vi "Camera Main.vi"(8 "Timeout 2":refnum<vi>, 9 "Main Open and Save Ctrls Ref":refnum<vi>[](array[refnum]), 11 "Camera":string) -> ()   [LabVIEW 2025]
uses:
  Camera Set Up/Ctrl/White Balance.ctl
  <vilib>/Utility/sysdir.llb/System Directory Type.ctl
  Main State Machine/Ctrl's/Main Cluster.ctl
  Main State Machine/Ctrl's/Main Queue.ctl
  Main State Machine/Ctrl's/Main States.ctl
  <vilib>/userDefined/High Color/IMAQdx.ctl
  <vilib>/vision/Image Controls.llb/IMAQ Image.ctl
  Camera Set Up/Event/Event Setup Types.ctl
  41b0be78-b641-410b-9a45-cddc263d6dc9.vi
  <vilib>/Utility/config.llb/Read Key (String).vi
  <vilib>/Utility/config.llb/Write Key (String).vi
  <vilib>/regexp/Match Regular Expression.xnode
  <vilib>/vision/driver/NI_Vision_Acquisition_Software.lvlib
  <vilib>/Utility/config.llb/NI_LVConfig.lvlib
  <resource>/objmgr/imaqdx.rc
  <vilib>/vision/NI_Vision_Development_Module.lvlib
panel:
  in  "Main":enum32{"Camera Settings", "Camera Settings 2"}(tab)
  out "Title":string="cam0"
  out "Greyscale":bool
  out "Camera Image":T1(plugin-control)
  in  "Save 2":bool caption="Save"
  in  "Reset Camera":bool
  in  "VideoMode":u16(ring)=20 items=["640x360 MJPG 260.00fps", "1280x720 MJPG 120.00fps", "1920x1080 MJPG 60.00fps"]
  in  "Saturation":i32(slide)=50 min=0 max=100 scale=0.0..100.0
  in  "Hue":i32(slide)=50 min=0 max=100 scale=0.0..100.0
  in  "Gamma":i32(slide)=50 min=0 max=100 scale=0.0..100.0
  in  "Exposure":dbl(slide)=2.0 min=0.0 max=100.0 step=0.01 scale=0.0..100.0
  in  "Contrast":i32(slide)=50 min=0 max=100 scale=0.0..100.0
  in  "Sharpness":i32(slide)=50 min=0 max=100 scale=0.0..100.0
  in  "White Balance":T2=enum."Hold current"
  in  "Gain":i32(slide)=50 min=0 max=100 scale=0.0..100.0
  in  "Brightness":i32(slide)=50 min=0 max=100 scale=0.0..100.0
  out "Width 2":u32=640 caption="Width"
  out "Height 2":u32=360 caption="Height"
  out "Processed FPS":dbl format="%.1f"
  out "Acquired FPS":dbl format="%.1f"
  out "Timeout":u32
  out "Running":bool
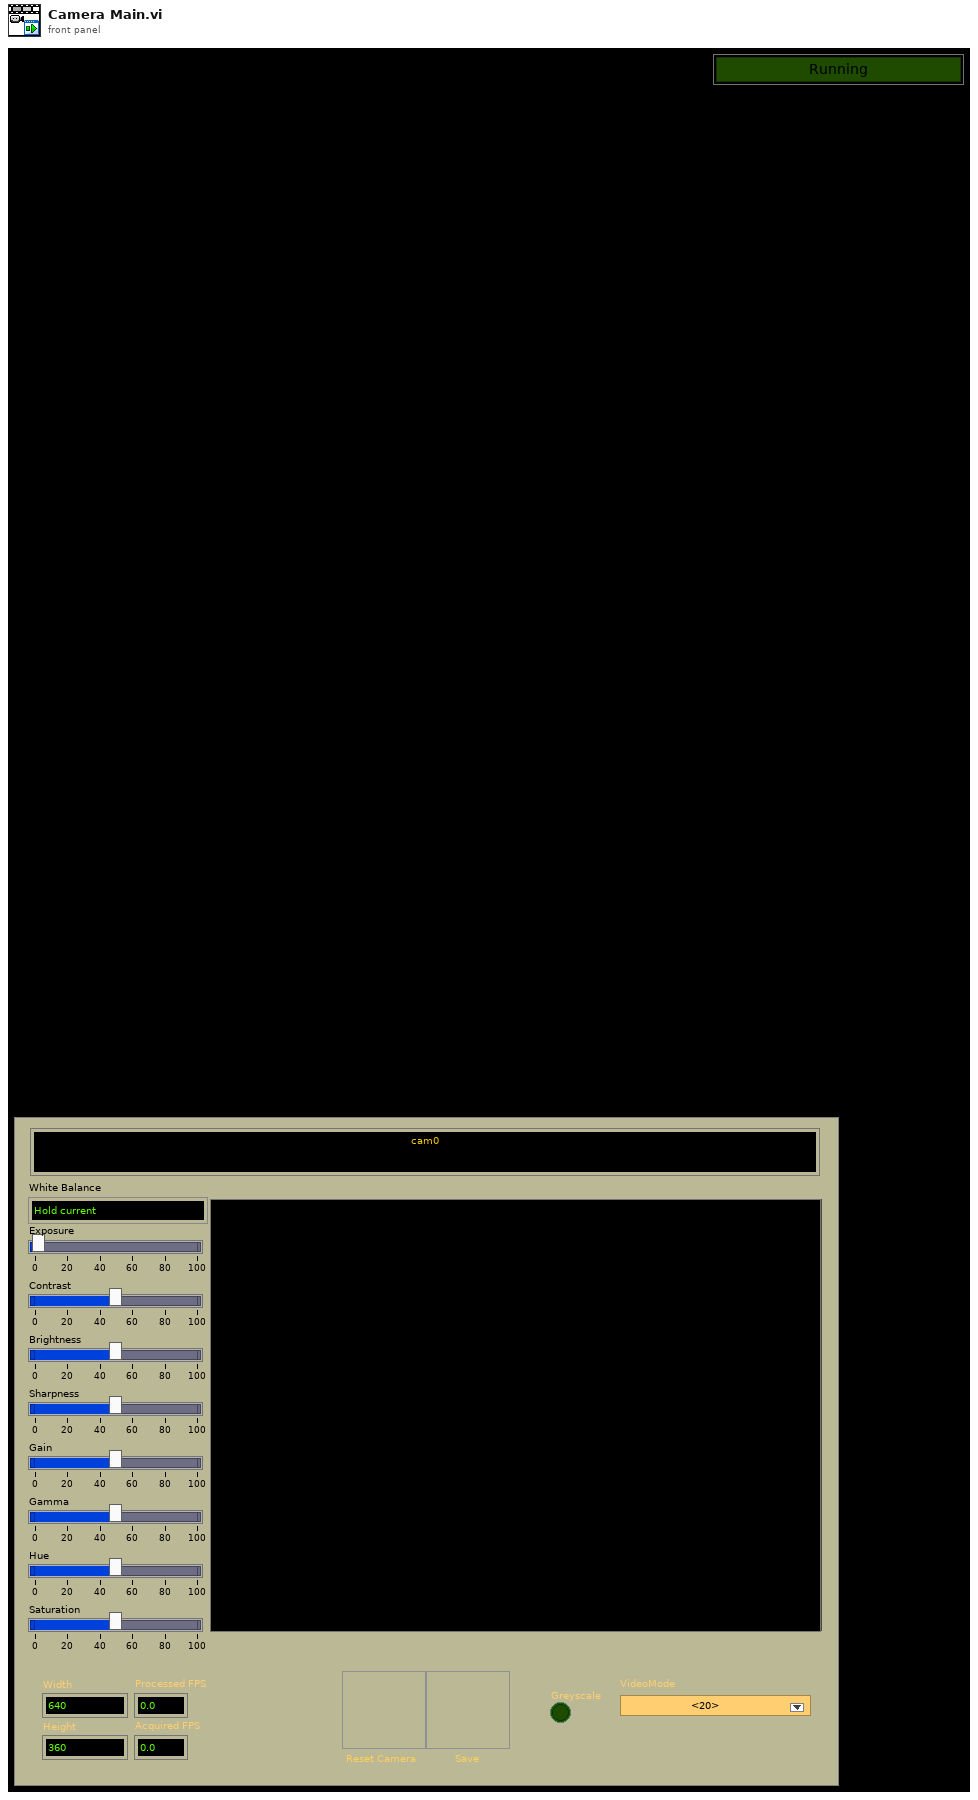
[diagram p1: front panel]
types:
  T1 = typedef "IMAQ Image.ctl" = refnum<image>
  T2 = typedef "White Balance.ctl" = enum16{"Auto", "Fixed indoor", "Fixed outdoor 1", "Fixed outdoor 2", "Fixed fluorescent 1", "Fixed fluorescent 2", "Hold current", "Custom"}
  T3 = typedef "System Directory Type.ctl" = i32
  T4 = typedef "Image Type" = u32
  T5 = typedef "Main Cluster.ctl" = cluster{"Main Queue":T6, "error":errorcluster, "Camera":T8, "Camera Session":T8, "Image In":T1, "White Balance":T2, "Attr String":string[], "Values":dbl[], "VideoMode":u16, "Exposure":i32, "Reset":bool, "Greyscale":bool, "INI path":path, "Default path":path, "INI File Found":bool, "Open And Save Controls":refnum<vi>[], "Buffer":u32, "Main Timeout ref":refnum<vi>, "Main Open and Save Ctrls Ref":refnum<vi>[]}
  T6 = typedef "Main Queue.ctl" = T7[]
  T7 = typedef "Main States.ctl" = enum16{"Message Dispatcher", "INI", "End Session", "Camera Process Settings", "Camera Open Default", "Camera Save Default", "Get Values", "Get VideoMode", "Open Camera", "Open Settings", "Save Settings", "Set Value", "Set VideoMode", "Set WB", "Setup Camera", "Start Session", "Exit"}
  T8 = typedef "IMAQdx.ctl" = refnum<k21>
  T9 = typedef "Event Setup Types.ctl" = enum16{"Default", "Camera Loop Started", "GreyScale", "Reset Camera Settings", "Reset Team Number", "Save Data", "Setting Changed", "Update Video Mode", "Video Mode Changed", "Exit"}
  T10 = enum8{"Enabled", "Disabled", "Disabled and Grayed Out"}
  T11 = typedef "NI_LVConfig.lvlib/Config Data RefNum.ctl" = refnum<k1>
  T12 = cluster{"Video Mode":u32, "Video Mode Name":string}[]
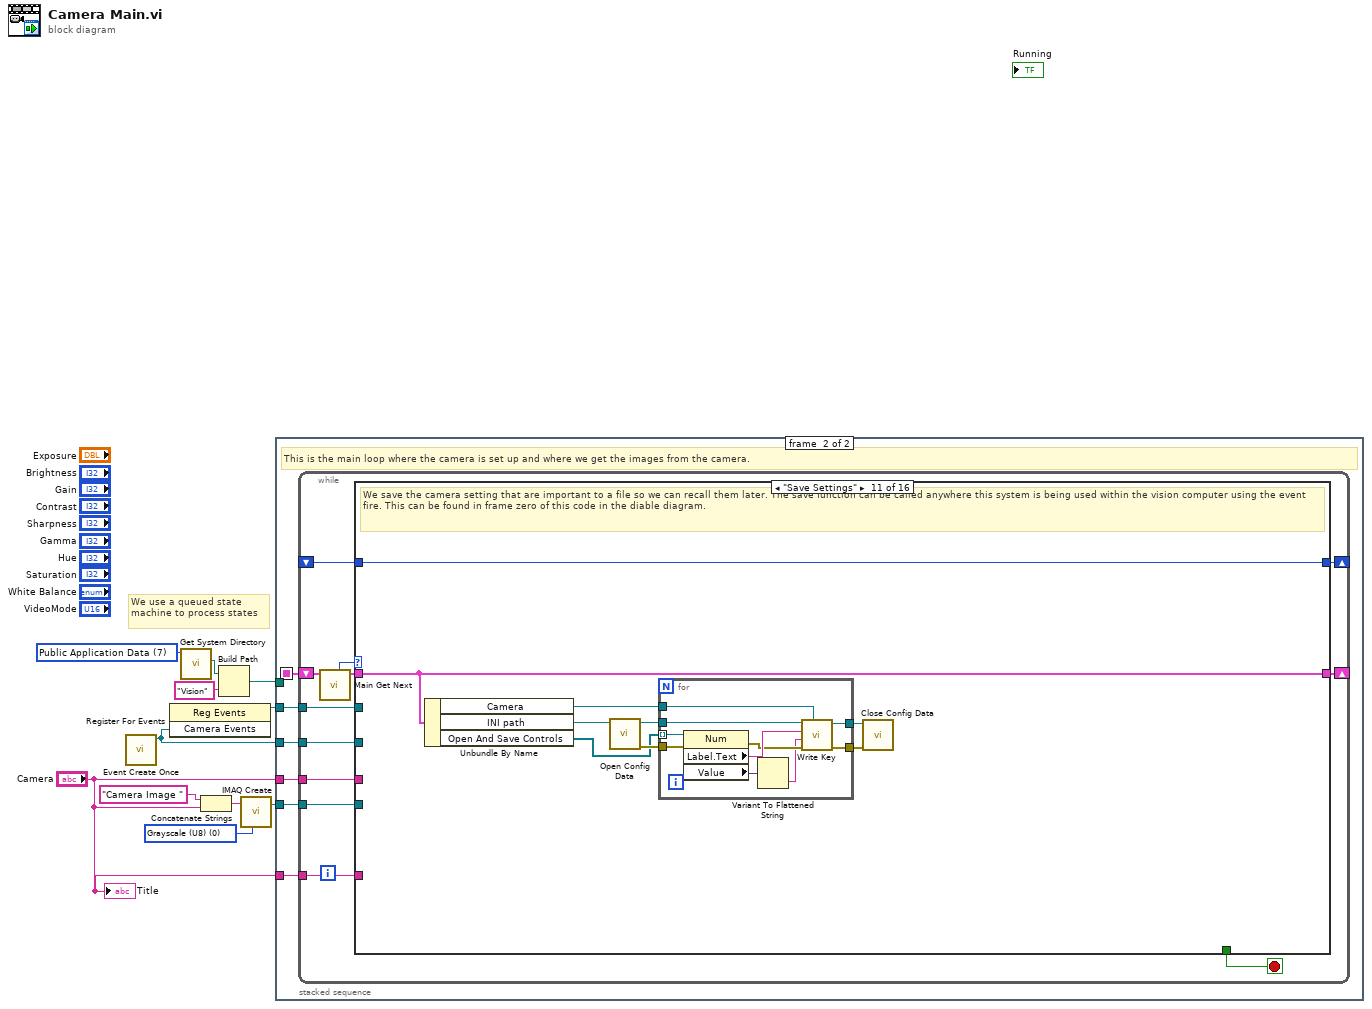
[diagram p0: block diagram]
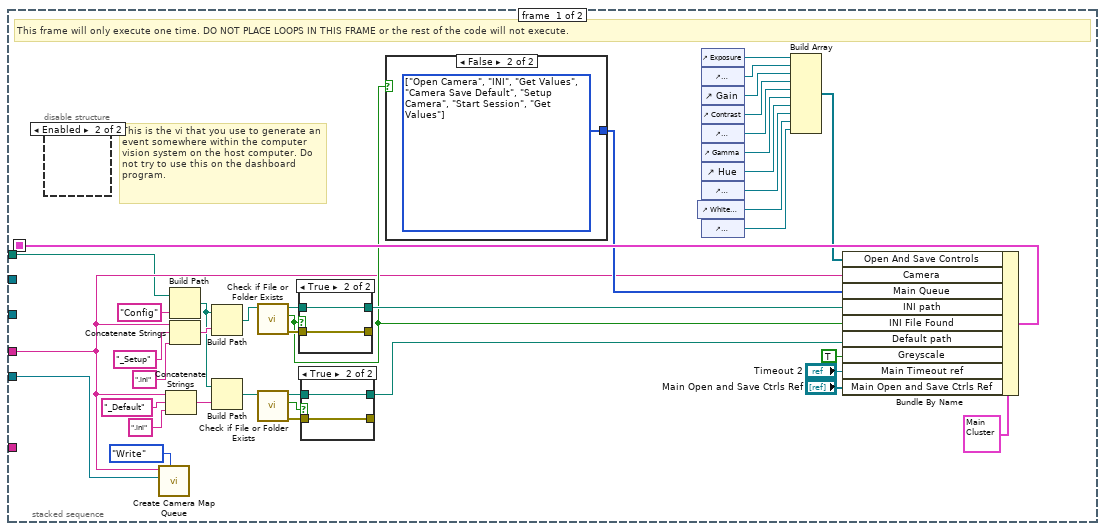
[diagram p2: hidden frame]
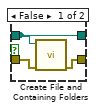
[diagram p3: hidden frame]
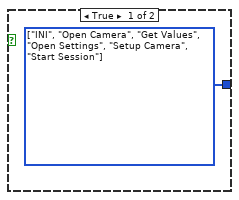
[diagram p4: hidden frame]
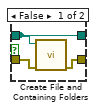
[diagram p5: hidden frame]
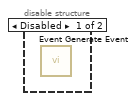
[diagram p6: hidden frame]
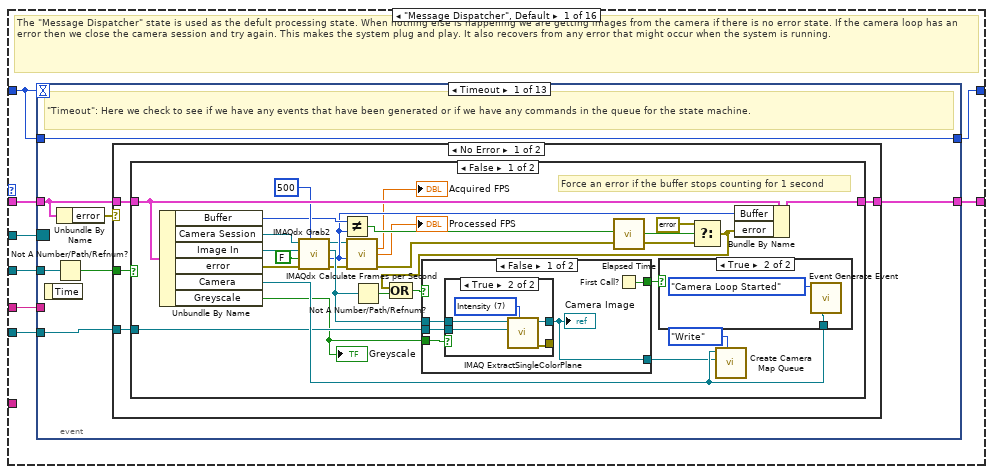
[diagram p7: hidden frame]
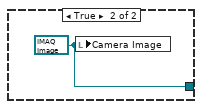
[diagram p10: hidden frame]
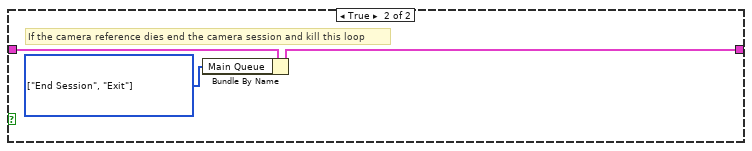
[diagram p11: hidden frame]
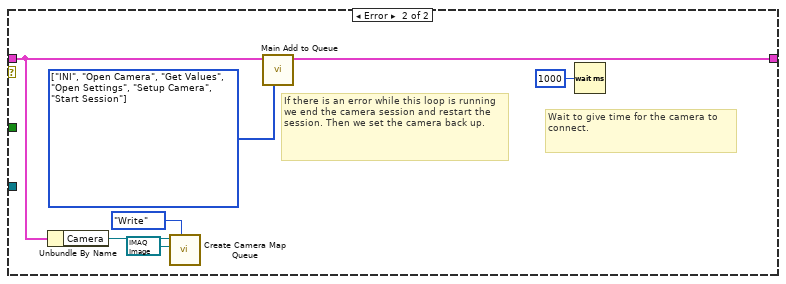
[diagram p12: hidden frame]
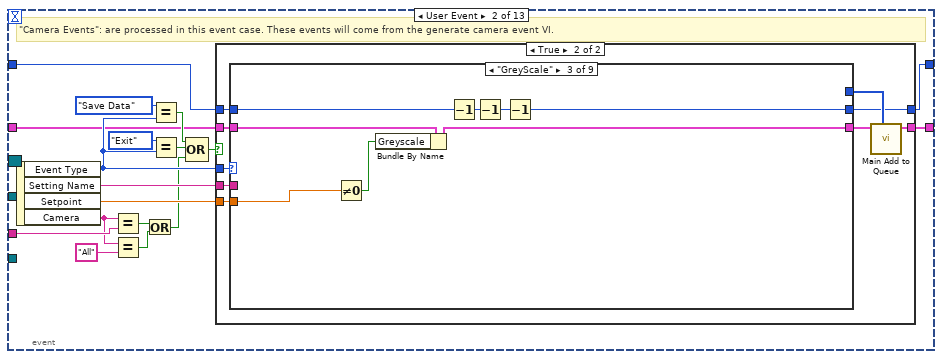
[diagram p13: hidden frame]
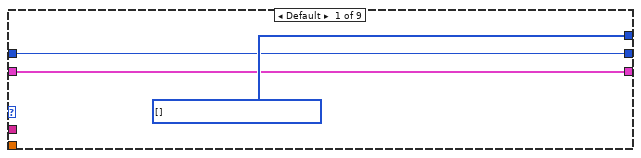
[diagram p15: hidden frame]
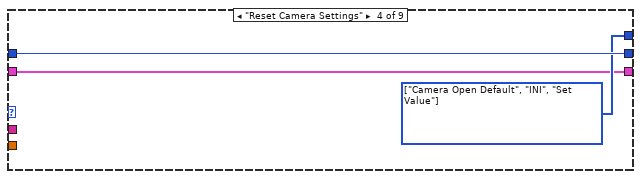
[diagram p17: hidden frame]
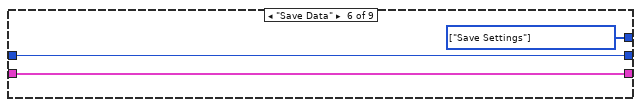
[diagram p19: hidden frame]
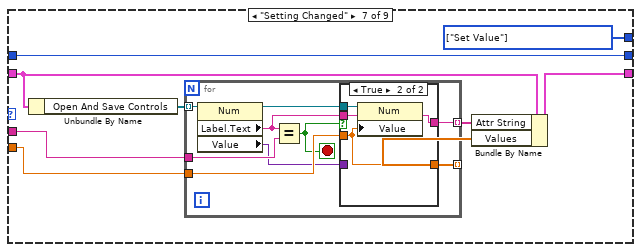
[diagram p20: hidden frame]
diagram:
  w5 = T3 7 items=["User Home"=0, "User Desktop"=1, "User Documents"=2, "User Application Data"=3, "User Preferences"=4, "User Temporary"=5, "Public Documents"=6, "Public Application Data"=7, "Public Preferences"=8, "Public Cache"=13, "System Core Libraries"=9, "System Installed Libraries"=10, "Application Files"=11, "Boot Volume Root"=12] ("system directory type")
  w8 = T4 0 items=["Grayscale (U8)", "Grayscale (I16)", "Grayscale (SGL)", "Complex (CSG)", "RGB (U32)", "HSL (U32)", "RGB (U64)", "Grayscale (U16)"] ("Image Type")
  # "We use a queued state machine to process states"
  n1 = call "Event Create Once.vi"() -> ("Camera Events"=w6:refnum<user-event>)  [unwired: 10 in, 1 out]
  n2 = register-events(w6) -> (reference out=w11:refnum<event-registration>)  [unwired: 2 in, 1 out]
  n3 = call <vilib>:"Get System Directory.vi"("system directory type"=w5) -> ("system directory"=w4:path)  [unwired: 10 in]
  n4 = Concatenate Strings("Camera Image " ("string"), "Camera") -> (w10:string)
  n5 = Build Path(base path=w4, name or relative path="Vision") -> (appended path=w3:path)
  n6 = call "IMAQ Create"("Image Name"=w10, "Image Type"=w8) -> ("New Image"=w7:T1)  [unwired: 2 in, 2 out]
  n7 = stacked-sequence {
    seq-local: [w46 _] -> [_ w68]
    tunnel: w11 -> [_ w67]
    tunnel: w6 -> [_ w66]
    tunnel: "Camera" -> [w25 w65]
    tunnel: w7 -> [w26 w64]
    tunnel: w3 -> [w13 _]
    tunnel: "Camera" -> [_ w63]
    frame #0 {
      # "This is the vi that you use to generate an event somewhere within the computer vision system on the host computer. Do not try to use this on the dashboard program."
      # "This frame will only execute one time. DO NOT PLACE LOOPS IN THIS FRAME or the rest of the code will not execute."
      n8 = disable-structure shown="Enabled" {
        frame Disabled {
          n9 = call "Event Generate Event.vi"() -> ()  [unwired: 12 in]
        }
        frame Enabled {
        }
      }
      n10 = call "Create Camera Map Queue.vi"("Action"=enum16{"Read", "Write"}."Write", "Image in"=w26, "Camera"=w25) -> ()  [unwired: 7 in, 2 out]
      n11 = Concatenate Strings(w25, "_Default" ("string"), ".ini" ("name or relative path")) -> (w28:string)
      n12 = Build Path(base path=w13, name or relative path="Config") -> (appended path=w31:path)
      n13 = Concatenate Strings(w25, "_Setup" ("string"), ".ini" ("name or relative path")) -> (w49:string)
      n14 = Build Path(base path=w31, name or relative path=w49) -> (appended path=w44:path)
      n15 = Build Path(base path=w31, name or relative path=w28) -> (appended path=w33:path)
      n16 = call <vilib>:"Check if File or Folder Exists.vi"("path"=w44) -> ("error out"=w45:errorcluster, "file or folder exists?"=w37:bool, "dup path"=w43:path)  [unwired: 8 in]
      n17 = call <vilib>:"Check if File or Folder Exists.vi"("path"=w33) -> ("error out"=w36:errorcluster, "file or folder exists?"=w34:bool, "dup path"=w35:path)  [unwired: 8 in]
      n18 = case shown="True" w37 {
        tunnel: [w60 w61] -> _
        tunnel: w45 -> [w59 w61]
        tunnel: w43 -> [w58 w62]
        tunnel: [w58 w62] -> w42
        frame False {
          n19 = call <vilib>:"Create File and Containing Folders.vi"("error in (no error)"=w59, "file path"=w58) -> ("error out"=w60:errorcluster)  [unwired: 8 in, 1 out]
        }
        frame True {
        }
      }
      n20 = case shown="True" w34 {
        tunnel: [w53 w54] -> _
        tunnel: w36 -> [w52 w54]
        tunnel: w35 -> [w51 w55]
        tunnel: [w51 w55] -> w32
        frame False {
          n21 = call <vilib>:"Create File and Containing Folders.vi"("error in (no error)"=w52, "file path"=w51) -> ("error out"=w53:errorcluster)  [unwired: 8 in, 1 out]
        }
        frame True {
        }
      }
      n22 = case shown="False" w37 {
        tunnel: [w56 w57] -> w38
        frame True {
          w56 = T6 [enum."INI", enum."Open Camera", enum."Get Values", enum."Open Settings", enum."Setup Camera", enum."Start Session"] items=["Message Dispatcher", "INI", "End Session", "Camera Process Settings", "Camera Open Default", "Camera Save Default", "Get Values", "Get VideoMode", "Open Camera", "Open Settings", "Save Settings", "Set Value", "Set VideoMode", "Set WB", "Setup Camera", "Start Session", "Exit"] ("Main Queue")
        }
        frame False {
          w57 = T6 [enum."Open Camera", enum."INI", enum."Get Values", enum."Camera Save Default", enum."Setup Camera", enum."Start Session", enum."Get Values"] items=["Message Dispatcher", "INI", "End Session", "Camera Process Settings", "Camera Open Default", "Camera Save Default", "Get Values", "Get VideoMode", "Open Camera", "Open Settings", "Save Settings", "Set Value", "Set VideoMode", "Set WB", "Setup Camera", "Start Session", "Exit"] ("Main Queue")
        }
      }
      n23 = control-ref of="White Balance"() -> (w15:refnum<vi>)
      n24 = control-ref of="Exposure"() -> (w23:refnum<vi>)
      n25 = control-ref of="Brightness"() -> (w22:refnum<vi>)
      n26 = control-ref of="Gain"() -> (w21:refnum<vi>)
      n27 = control-ref of="Contrast"() -> (w20:refnum<vi>)
      n28 = control-ref of="Sharpness"() -> (w19:refnum<vi>)
      n29 = control-ref of="Gamma"() -> (w18:refnum<vi>)
      n30 = control-ref of="Hue"() -> (w17:refnum<vi>)
      n31 = control-ref of="Saturation"() -> (w16:refnum<vi>)
      n32 = control-ref of="VideoMode"() -> (w14:refnum<vi>)
      n33 = Build Array(w23, w22, w21, w20, w19, w18, w17, w16, w15, w14) -> (w41:refnum<vi>[])
      n34 = Bundle By Name(cluster=T5 {"Main Queue"=[], "error"={"status"=FALSE, "code"=0, "source"=""}, "Camera"="", "Camera Session"="", "Image In"=refnum, "White Balance"=enum."Hold current", "Attr String"=[], "Values"=[], "VideoMode"=0, "Exposure"=50, "Reset"=FALSE, "Greyscale"=FALSE, "INI path"=path "", "Default path"=path "", "INI File Found"=FALSE, "Open And Save Controls"=[], "Buffer"=0, "Main Timeout ref"=refnum, "Main Open and Save Ctrls Ref"=[]} ("Main Cluster Out"), "Open And Save Controls"=w41, "Camera"=w25, "Main Queue"=w38, "INI path"=w42, "INI File Found"=w37, "Default path"=w32, "Greyscale"=TRUE, "Main Timeout ref"="Timeout 2", "Main Open and Save Ctrls Ref"="Main Open and Save Ctrls Ref") -> (w46:T5)
    }
    frame #1 {
      # "This is the main loop where the camera is set up and where we get the images from the camera."
      n35 = while {
        shift-right: [w76] -> _
        shift-left: w68 -> [w78]
        tunnel: w67 -> [w75]
        shift-right: [w74] -> _
        shift-left: _ -> [w73]
        tunnel: w66 -> [w72]
        tunnel: w65 -> [w71]
        tunnel: w64 -> [w70]
        tunnel: w63 -> [w69]
        stop <- w80 stop-if-true
        n36 = call "Main Get Next.vi"("Main Cluster In"=w78) -> ("Main Cluster Out"=w77:T5, "Next State"=w79:T7)  [unwired: 9 in]
        n37 = case shown="\"Save Settings\"" w79 {
          tunnel: [_ _ _ _ _ _ _ _ _ _ _ _ _ _ _ TRUE] -> w80
          tunnel: w77 -> [w87 w327 w339 w347 w390 w395 w417 w465 w591 w610 w658 w677 w695 w754 w890 w899]
          tunnel: [w88 w328 w336 w344 w388 w395 w416 w464 w590 w606 w658 w676 w705 w752 w884 w899] -> w76
          tunnel: w75 -> [w86 _ _ _ _ _ _ _ _ _ _ _ _ _ _ _]
          tunnel: w73 -> [w84 w330 w337 w351 w389 w400 w422 _ w596 w614 w663 w683 w694 _ w887 w897]
          tunnel: [w83 w330 w337 w351 w389 w400 w422 w439 w596 w614 w663 w683 w694 w728 w887 w897] -> w74
          tunnel: w72 -> [w85 _ _ _ _ _ _ _ _ _ _ _ _ _ _ _]
          tunnel: w71 -> [w82 _ _ _ _ _ _ _ _ _ _ _ _ _ _ _]
          tunnel: w70 -> [w81 _ _ _ _ _ _ _ _ _ _ _ _ _ _ _]
          tunnel: w69 -> [_ _ _ _ _ _ _ _ w585 _ _ _ _ _ _ _]
          frame "Message Dispatcher", Default {
            # "The \"Message Dispatcher\" state is used as the defult processing state. When nothing else is happening we are getting images from the camera if there is no error state. If the camera loop has an error then we close the camera session and try again. This makes the system plug and play. It also recovers from any error that might occur when the system is running."
            n38 = event shown="[0] Timeout" {
              selector: w86 -> [_ _ _ _ _ _ _ _ _ _ _ _ _]
              dyn-events: _ -> [_ _ _ _ _ _ _ _ _ _ _ _ _]
              timeout: w84 -> [_ _ _ _ _ _ _ _ _ _ _ _ _]
              tunnel: [w95 w168 w240 w250 w260 w270 w280 w284 w291 w298 w308 w314 w323] -> w88
              tunnel: w87 -> [w94 w161 w242 w252 w262 w272 w282 w287 w290 w300 w310 w316 w325]
              tunnel: w85 -> [w92 _ _ _ _ _ _ _ _ _ _ _ _]
              tunnel: w84 -> [w90 w160 w234 w244 w254 w264 w274 w285 w288 w292 w302 w312 w321]
              tunnel: [w90 w159 w234 w244 w254 w264 w274 w285 w288 w292 w302 w312 w321] -> w83
              tunnel: w82 -> [_ w158 _ _ _ _ _ _ _ _ _ _ _]
              tunnel: w81 -> [w89 _ _ _ _ _ _ _ _ _ _ _ _]
              event Timeout {
                # "\"Timeout\": Here we check to see if we have any events that have been generated or if we have any commands in the queue for the state machine."
                n39 = event-data() -> ()  [unwired: 1 in, 1 out]
                n40 = Not A Number/Path/Refnum?(number/path/refnum=w92) -> (NaN/Path/Refnum?=w91:bool)
                n41 = Unbundle By Name(w94) -> ("error"=w93:errorcluster)
                n42 = case shown="No Error" w93 {
                  tunnel: w94 -> [w99 w147]
                  tunnel: [w98 w150] -> w95
                  tunnel: w91 -> [w97 _]
                  tunnel: w89 -> [w96 _]
                  frame No Error {
                    n43 = case shown="False" w97 {
                      tunnel: w99 -> [w126 w143]
                      tunnel: [w121 w142] -> w98
                      tunnel: w96 -> [w119 _]
                      frame False {
                        # "Force an error if the buffer stops counting for 1 second"
                        n44 = Unbundle By Name(w126) -> ("Buffer"=w107:u32, "Camera Session"=w106:T8, "Image In"=w125:T1, "error"=w124:errorcluster, "Camera"=w122:T8, "Greyscale"=w118:bool)
                        "Greyscale" <- w118
                        n45 = call <vilib>:"IMAQdx Grab2.vi"("Timeout (ms)"=500, "error in"=w124, "Wait for Next Buffer? (Yes)"=FALSE, "Image In"=w125, "Session In"=w106) -> ("error out"=w102:errorcluster, "Buffer Number Out"=w105:u32, "Image Out"=w114:T1, "Session Out"=w100:T8)  [unwired: 3 in]
                        n46 = Not Equal?(x=w107, y=w105) -> (x != y?=w116:bool)
                        n47 = call <vilib>:"IMAQdx Calculate Frames per Second.vi"("Session In"=w100, "Buffer Number"=w105, "error in (no error)"=w102) -> ("Acquired Frames per Second"=→"Acquired FPS":dbl, "Processed Frames per Second"=→"Processed FPS":dbl, "error out"=w101:errorcluster)  [unwired: 6 in, 4 out]
                        n48 = Not A Number/Path/Refnum?(number/path/refnum=w114) -> (NaN/Path/Refnum?=w113:bool)
                        n49 = call "Elapsed Time"("Reset"=w116) -> ("Time has Elapsed"=w115:bool)  [unwired: 11 in, 7 out]
                        n50 = Select(t=errorcluster {"status"=TRUE, "code"=1, "source"=""}, s=w115, f=w101) -> (s? t:f=w112:errorcluster)
                        n51 = Compound Arithmetic op=OR(w112, w113) -> (w111:bool)
                        n52 = case shown="False" w111 {
                          tunnel: w114 -> [w132 _]
                          tunnel: [w133 _] -> w123
                          tunnel: w119 -> [w131 _]
                          tunnel: w118 -> [w130 _]
                          tunnel: [w129 w140] -> w109
                          frame False {
                            n53 = case shown="True" w130 {
                              tunnel: w132 -> [w134 w139]
                              tunnel: [w134 w138] -> w129
                              tunnel: w131 -> [_ w136]
                              tunnel: [_ w135] -> _
                              frame False {
                              }
                              frame True {
                                w137 = 7 items=["Red", "Green", "Blue", "Hue", "Saturation", "Luminance", "Value", "Intensity"] ("Color Plane")
                                n54 = call "IMAQ ExtractSingleColorPlane"("Color Plane"=w137, "Image Dst"=w136, "Image Src"=w139) -> ("error out"=w135:errorcluster, "Image Dst Out"=w138:T1)  [unwired: 7 in]
                              }
                            }
                            "Camera Image" <- w129
                            n55 = First Call?() -> (First Call?: T/F=w133:bool)
                          }
                          frame True {
                            w140 = T1 refnum ("Camera Image")
                            n56 = local write "Camera Image"(w140) -> ()
                          }
                        }
                        n57 = case shown="True" w123 {
                          tunnel: w122 -> [_ w127]
                          frame False {
                          }
                          frame True {
                            n58 = call "Event Generate Event.vi"("Camera Name"=w127, "Event Type"=Event_Setup_Types."Camera Loop Started") -> ()  [unwired: 10 in]
                          }
                        }
                        n59 = call "Create Camera Map Queue.vi"("Action"=enum16{"Read", "Write"}."Write", "Image in"=w109, "Camera"=w122) -> ()  [unwired: 7 in, 2 out]
                        n60 = Bundle By Name(cluster=w126, "Buffer"=w105, "error"=w112) -> (w121:T5)
                      }
                      frame True {
                        w141 = T6 [enum."End Session", enum."Exit"] items=["Message Dispatcher", "INI", "End Session", "Camera Process Settings", "Camera Open Default", "Camera Save Default", "Get Values", "Get VideoMode", "Open Camera", "Open Settings", "Save Settings", "Set Value", "Set VideoMode", "Set WB", "Setup Camera", "Start Session", "Exit"] ("Main Queue")
                        # "If the camera reference dies end the camera session and kill this loop"
                        n61 = Bundle By Name(cluster=w143, "Main Queue"=w141) -> (w142:T5)
                      }
                    }
                  }
                  frame Error {
                    w144 = T6 [enum."INI", enum."Open Camera", enum."Get Values", enum."Open Settings", enum."Setup Camera", enum."Start Session"] items=["Message Dispatcher", "INI", "End Session", "Camera Process Settings", "Camera Open Default", "Camera Save Default", "Get Values", "Get VideoMode", "Open Camera", "Open Settings", "Save Settings", "Set Value", "Set VideoMode", "Set WB", "Setup Camera", "Start Session", "Exit"] ("Main Queue")
                    # "Wait to give time for the camera to connect."
                    # "If there is an error while this loop is running we end the camera session and restart the session. Then we set the camera back up."
                    n62 = Unbundle By Name(w147) -> ("Camera"=w146:T8)
                    n63 = call "Create Camera Map Queue.vi"("Action"=enum16{"Read", "Write"}."Write", "Image in"=T1 refnum, "Camera"=w146) -> ()  [unwired: 7 in, 2 out]
                    n64 = call "Main Add to Queue.vi"("Main Queue"=w144, "Main Cluster In"=w147) -> ("Main Cluster Out"=w150:T5)  [unwired: 9 in]
                    n65 = Wait (ms)(milliseconds to wait=u32 1000) -> ()  [unwired: 1 out]
                  }
                }
              }
              event User Event {
                # "\"Camera Events\": are processed in this event case. These events will come from the generate camera event VI."
                n66 = event-data() -> ("Event Type"=w162:T9, "Setting Name"=w157:string, "Setpoint"=w156:dbl, "Camera"=w153:string)  [unwired: 1 in]
                n67 = Equal?(x=w153, y=w158) -> (x = y?=w154:bool)
                n68 = Equal?(x=w153, y="All") -> (x = y?=w151:bool)
                n69 = Or(x=w154, y=w151) -> (x .or. y?=w155:bool)
                n70 = Equal?(x=Event_Setup_Types."Save Data", y=w162) -> (x = y?=w163:bool)
                n71 = Equal?(x=Event_Setup_Types."Exit", y=w162) -> (x = y?=w166:bool)
                n72 = Compound Arithmetic op=OR(w163, w166, w155) -> (w165:bool)
                n73 = case shown="True" w165 {
                  tunnel: w161 -> [w170 w175]
                  tunnel: [w170 w176] -> w168
                  tunnel: w156 -> [_ w179]
                  tunnel: w162 -> [_ w177]
                  tunnel: w160 -> [w169 w174]
                  tunnel: [w169 w173] -> w159
                  tunnel: w157 -> [_ w171]
                  frame False {
                  }
                  frame True {
                    n74 = case shown="\"GreyScale\"" w177 {
                      tunnel: w179 -> [_ _ w190 _ _ _ w203 w229 _]
                      tunnel: [w182 _ _ w194 _ w198 w205 w228 w233] -> w178
                      tunnel: w175 -> [w181 w183 w192 w193 w196 w199 w207 w227 w232]
                      tunnel: w174 -> [w180 w184 w188 w195 w197 w200 w209 w230 w231]
                      tunnel: [w180 w184 w185 w195 w197 w200 w209 w230 w231] -> w173
                      tunnel: [w181 w183 w191 w193 w196 w199 w206 w226 w232] -> w172
                      tunnel: w171 -> [_ _ _ _ _ _ w204 _ _]
                      frame Default {
                        w182 = T6 [] items=["Message Dispatcher", "INI", "End Session", "Camera Process Settings", "Camera Open Default", "Camera Save Default", "Get Values", "Get VideoMode", "Open Camera", "Open Settings", "Save Settings", "Set Value", "Set VideoMode", "Set WB", "Setup Camera", "Start Session", "Exit"] ("Main Queue")
                      }
                      frame "Camera Loop Started" {
                      }
                      frame "GreyScale" {
                        n75 = Not Equal To 0?(x=w190) -> (x != 0?=w189:bool)
                        n76 = Bundle By Name(cluster=w192, "Greyscale"=w189) -> (w191:T5)
                        n77 = Decrement(x=w188) -> (x-1=w187:u32)
                        n78 = Decrement(x=w187) -> (x-1=w186:u32)
                        n79 = Decrement(x=w186) -> (x-1=w185:u32)
                      }
                      frame "Reset Camera Settings" {
                        w194 = T6 [enum."Camera Open Default", enum."INI", enum."Set Value"] items=["Message Dispatcher", "INI", "End Session", "Camera Process Settings", "Camera Open Default", "Camera Save Default", "Get Values", "Get VideoMode", "Open Camera", "Open Settings", "Save Settings", "Set Value", "Set VideoMode", "Set WB", "Setup Camera", "Start Session", "Exit"] ("Main Queue")
                      }
                      frame "Reset Team Number" {
                      }
                      frame "Save Data" {
                        w198 = T6 [enum."Save Settings"] items=["Message Dispatcher", "INI", "End Session", "Camera Process Settings", "Camera Open Default", "Camera Save Default", "Get Values", "Get VideoMode", "Open Camera", "Open Settings", "Save Settings", "Set Value", "Set VideoMode", "Set WB", "Setup Camera", "Start Session", "Exit"] ("Main Queue")
                      }
                      frame "Setting Changed" {
                        w205 = T6 [enum."Set Value"] items=["Message Dispatcher", "INI", "End Session", "Camera Process Settings", "Camera Open Default", "Camera Save Default", "Get Values", "Get VideoMode", "Open Camera", "Open Settings", "Save Settings", "Set Value", "Set VideoMode", "Set WB", "Setup Camera", "Start Session", "Exit"] ("Main Queue")
                        n80 = Unbundle By Name(w207) -> ("Open And Save Controls"=w208:refnum<vi>[])
                        n81 = for {
                          tunnel: w204 -> [w217]
                          tunnel: w203 -> [w216]
                          tunnel: [w210] -> w202 mode=indexing
                          tunnel: w208 -> [w218] mode=indexing
                          tunnel: [w212] -> w201 mode=indexing
                          stop <- w214 stop-if-true
                          n82 = property class="Num"(reference=w218) -> (reference out=w215:refnum<vi>, "Label.Text"=w211:string, "Value"=w213:variant)  [unwired: 1 in, 1 out]
                          n83 = Equal?(x=w211, y=w217) -> (x = y?=w214:bool)
                          n84 = case shown="True" w214 {
                            tunnel: w216 -> [_ w224]
                            tunnel: w215 -> [_ w225]
                            tunnel: w213 -> [w221 _]
                            tunnel: [w219 w224] -> w212
                            tunnel: w211 -> [w222 w223]
                            tunnel: [w222 w223] -> w210
                            frame False {
                              n85 = Variant To Data(type=0.0, Variant=w221) -> (data=w219:dbl)  [unwired: 1 in, 1 out]
                            }
                            frame True {
                              n86 = property class="Num"(reference=w225, "Value"=w224) -> ()  [unwired: 1 in, 2 out]
                            }
                          }
                        }
                        n87 = Bundle By Name(cluster=w207, "Attr String"=w202, "Values"=w201) -> (w206:T5)
                      }
                      frame "Video Mode Changed" {
                        w228 = T6 [enum."End Session", enum."Open Camera", enum."Get Values", enum."Setup Camera", enum."Start Session", enum."Get Values"] items=["Message Dispatcher", "INI", "End Session", "Camera Process Settings", "Camera Open Default", "Camera Save Default", "Get Values", "Get VideoMode", "Open Camera", "Open Settings", "Save Settings", "Set Value", "Set VideoMode", "Set WB", "Setup Camera", "Start Session", "Exit"] ("Main Queue")
                        n88 = Bundle By Name(cluster=w227, "VideoMode"=w229) -> (w226:T5)
                        n89 = property on="VideoMode" class="Ring (strict)"("Value"=w229) -> ()  [unwired: 2 in, 2 out]
                      }
                      frame "Exit" {
                        w233 = T6 [enum."End Session", enum."Exit"] items=["Message Dispatcher", "INI", "End Session", "Camera Process Settings", "Camera Open Default", "Camera Save Default", "Get Values", "Get VideoMode", "Open Camera", "Open Settings", "Save Settings", "Set Value", "Set VideoMode", "Set WB", "Setup Camera", "Start Session", "Exit"] ("Main Queue")
                      }
                    }
                    n90 = call "Main Add to Queue.vi"("Main Queue"=w178, "Main Cluster In"=w172) -> ("Main Cluster Out"=w176:T5)  [unwired: 9 in]
                  }
                }
              }
              event "Brightness": Mouse Up {
                w241 = T6 [enum."Set Value"] items=["Message Dispatcher", "INI", "End Session", "Camera Process Settings", "Camera Open Default", "Camera Save Default", "Get Values", "Get VideoMode", "Open Camera", "Open Settings", "Save Settings", "Set Value", "Set VideoMode", "Set WB", "Setup Camera", "Start Session", "Exit"] ("Main Queue")
                # "Bringness: When the brigness is changed it fires this event to update the brightness."
                n91 = event-data() -> ("CtlRef"=w239:refnum<vi>)  [unwired: 1 in]
                n92 = property class="Slide (strict)"(reference=w239) -> ("Label.Text"=w237:string, "Value"=w238:i32)  [unwired: 1 in, 2 out]
                n93 = Build Array(w238) -> (w235:i32[])
                n94 = Build Array(w237) -> (w236:string[])
                n95 = call "Main Add to Queue.vi"("Main Queue"=w241, "Main Cluster In"=w242) -> ("Main Cluster Out"=w243:T5)  [unwired: 9 in]
                n96 = Bundle By Name(cluster=w243, "Attr String"=w236, "Values"=w235) -> (w240:T5)
              }
              event "Contrast": Mouse Up {
                w251 = T6 [enum."Set Value"] items=["Message Dispatcher", "INI", "End Session", "Camera Process Settings", "Camera Open Default", "Camera Save Default", "Get Values", "Get VideoMode", "Open Camera", "Open Settings", "Save Settings", "Set Value", "Set VideoMode", "Set WB", "Setup Camera", "Start Session", "Exit"] ("Main Queue")
                # "Camera Exposure: This is the array of states that are required to changed the exposure on the camera. This may be different for every USB camera model."
                n97 = event-data() -> ("CtlRef"=w249:refnum<vi>)  [unwired: 1 in]
                n98 = property class="Slide (strict)"(reference=w249) -> ("Label.Text"=w246:string, "Value"=w248:i32)  [unwired: 1 in, 2 out]
                n99 = Build Array(w246) -> (w245:string[])
                n100 = Build Array(w248) -> (w247:i32[])
                n101 = call "Main Add to Queue.vi"("Main Queue"=w251, "Main Cluster In"=w252) -> ("Main Cluster Out"=w253:T5)  [unwired: 9 in]
                n102 = Bundle By Name(cluster=w253, "Attr String"=w245, "Values"=w247) -> (w250:T5)
              }
              event "Exposure": Mouse Up {
                w261 = T6 [enum."Set Value"] items=["Message Dispatcher", "INI", "End Session", "Camera Process Settings", "Camera Open Default", "Camera Save Default", "Get Values", "Get VideoMode", "Open Camera", "Open Settings", "Save Settings", "Set Value", "Set VideoMode", "Set WB", "Setup Camera", "Start Session", "Exit"] ("Main Queue")
                # "Camera Exposure: This is the array of states that are required to changed the exposure on the camera. This may be different for every USB camera model."
                n103 = event-data() -> ("CtlRef"=w259:refnum<vi>)  [unwired: 1 in]
                n104 = property class="Slide (strict)"(reference=w259) -> ("Value"=w258:dbl, "Label.Text"=w256:string)  [unwired: 1 in, 2 out]
                n105 = Build Array(w258) -> (w257:dbl[])
                n106 = Build Array(w256) -> (w255:string[])
                n107 = call "Main Add to Queue.vi"("Main Queue"=w261, "Main Cluster In"=w262) -> ("Main Cluster Out"=w263:T5)  [unwired: 9 in]
                n108 = Bundle By Name(cluster=w263, "Values"=w257, "Attr String"=w255) -> (w260:T5)
              }
              event "Gamma": Mouse Up {
                w271 = T6 [enum."Set Value"] items=["Message Dispatcher", "INI", "End Session", "Camera Process Settings", "Camera Open Default", "Camera Save Default", "Get Values", "Get VideoMode", "Open Camera", "Open Settings", "Save Settings", "Set Value", "Set VideoMode", "Set WB", "Setup Camera", "Start Session", "Exit"] ("Main Queue")
                # "Save Settings: When this event is fired it will send the state to save the current settings to the setup file."
                n109 = event-data() -> ("CtlRef"=w269:refnum<vi>)  [unwired: 1 in]
                n110 = property class="Slide (strict)"(reference=w269) -> ("Value"=w268:i32, "Label.Text"=w267:string)  [unwired: 1 in, 2 out]
                n111 = Build Array(w268) -> (w265:i32[])
                n112 = Build Array(w267) -> (w266:string[])
                n113 = call "Main Add to Queue.vi"("Main Queue"=w271, "Main Cluster In"=w272) -> ("Main Cluster Out"=w273:T5)  [unwired: 9 in]
                n114 = Bundle By Name(cluster=w273, "Values"=w265, "Attr String"=w266) -> (w270:T5)
              }
              event "Hue": Mouse Up {
                w281 = T6 [enum."Set Value"] items=["Message Dispatcher", "INI", "End Session", "Camera Process Settings", "Camera Open Default", "Camera Save Default", "Get Values", "Get VideoMode", "Open Camera", "Open Settings", "Save Settings", "Set Value", "Set VideoMode", "Set WB", "Setup Camera", "Start Session", "Exit"] ("Main Queue")
                # "Save Settings: When this event is fired it will send the state to save the current settings to the setup file."
                n115 = event-data() -> ("CtlRef"=w279:refnum<vi>)  [unwired: 1 in]
                n116 = property class="Slide (strict)"(reference=w279) -> ("Value"=w278:i32, "Label.Text"=w277:string)  [unwired: 1 in, 2 out]
                n117 = Build Array(w278) -> (w275:i32[])
                n118 = Build Array(w277) -> (w276:string[])
                n119 = call "Main Add to Queue.vi"("Main Queue"=w281, "Main Cluster In"=w282) -> ("Main Cluster Out"=w283:T5)  [unwired: 9 in]
                n120 = Bundle By Name(cluster=w283, "Values"=w275, "Attr String"=w276) -> (w280:T5)
              }
              event "Reset Camera": Mouse Up {
                w286 = T6 [enum."Camera Open Default", enum."INI", enum."Set Value"] items=["Message Dispatcher", "INI", "End Session", "Camera Process Settings", "Camera Open Default", "Camera Save Default", "Get Values", "Get VideoMode", "Open Camera", "Open Settings", "Save Settings", "Set Value", "Set VideoMode", "Set WB", "Setup Camera", "Start Session", "Exit"] ("Main Queue")
                # "Save Settings: When this event is fired it will send the state to save the current settings to the setup file."
                n121 = event-data() -> ()  [unwired: 1 in, 1 out]
                n122 = call "Main Add to Queue.vi"("Main Queue"=w286, "Main Cluster In"=w287) -> ("Main Cluster Out"=w284:T5)  [unwired: 9 in]
              }
              event "Save 2": Mouse Up {
                w289 = T6 [enum."Save Settings"] items=["Message Dispatcher", "INI", "End Session", "Camera Process Settings", "Camera Open Default", "Camera Save Default", "Get Values", "Get VideoMode", "Open Camera", "Open Settings", "Save Settings", "Set Value", "Set VideoMode", "Set WB", "Setup Camera", "Start Session", "Exit"] ("Main Queue")
                # "Save Settings: When this event is fired it will send the state to save the current settings to the setup file."
                n123 = event-data() -> ()  [unwired: 1 in, 1 out]
                n124 = call "Main Add to Queue.vi"("Main Queue"=w289, "Main Cluster In"=w290) -> ("Main Cluster Out"=w291:T5)  [unwired: 9 in]
              }
              event "Sharpness": Mouse Up {
                w299 = T6 [enum."Set Value"] items=["Message Dispatcher", "INI", "End Session", "Camera Process Settings", "Camera Open Default", "Camera Save Default", "Get Values", "Get VideoMode", "Open Camera", "Open Settings", "Save Settings", "Set Value", "Set VideoMode", "Set WB", "Setup Camera", "Start Session", "Exit"] ("Main Queue")
                # "Save Settings: When this event is fired it will send the state to save the current settings to the setup file."
                n125 = event-data() -> ("CtlRef"=w297:refnum<vi>)  [unwired: 1 in]
                n126 = property class="Slide (strict)"(reference=w297) -> ("Value"=w296:i32, "Label.Text"=w295:string)  [unwired: 1 in, 2 out]
                n127 = Build Array(w296) -> (w293:i32[])
                n128 = Build Array(w295) -> (w294:string[])
                n129 = call "Main Add to Queue.vi"("Main Queue"=w299, "Main Cluster In"=w300) -> ("Main Cluster Out"=w301:T5)  [unwired: 9 in]
                n130 = Bundle By Name(cluster=w301, "Values"=w293, "Attr String"=w294) -> (w298:T5)
              }
              event "Saturation": Mouse Up {
                w309 = T6 [enum."Set Value"] items=["Message Dispatcher", "INI", "End Session", "Camera Process Settings", "Camera Open Default", "Camera Save Default", "Get Values", "Get VideoMode", "Open Camera", "Open Settings", "Save Settings", "Set Value", "Set VideoMode", "Set WB", "Setup Camera", "Start Session", "Exit"] ("Main Queue")
                # "Save Settings: When this event is fired it will send the state to save the current settings to the setup file."
                n131 = event-data() -> ("CtlRef"=w307:refnum<vi>)  [unwired: 1 in]
                n132 = property class="Slide (strict)"(reference=w307) -> ("Value"=w306:i32, "Label.Text"=w305:string)  [unwired: 1 in, 2 out]
                n133 = Build Array(w306) -> (w303:i32[])
                n134 = Build Array(w305) -> (w304:string[])
                n135 = call "Main Add to Queue.vi"("Main Queue"=w309, "Main Cluster In"=w310) -> ("Main Cluster Out"=w311:T5)  [unwired: 9 in]
                n136 = Bundle By Name(cluster=w311, "Values"=w303, "Attr String"=w304) -> (w308:T5)
              }
              event Value Change {
                w315 = T6 [enum."Set WB"] items=["Message Dispatcher", "INI", "End Session", "Camera Process Settings", "Camera Open Default", "Camera Save Default", "Get Values", "Get VideoMode", "Open Camera", "Open Settings", "Save Settings", "Set Value", "Set VideoMode", "Set WB", "Setup Camera", "Start Session", "Exit"] ("Main Queue")
                # "White Balance: when the whitebalance value is changed it will fire this event and cause the state to be added to the message queue."
                n137 = event-data() -> ("NewVal"=w313:T2)  [unwired: 1 in]
                n138 = call "Main Add to Queue.vi"("Main Queue"=w315, "Main Cluster In"=w316) -> ("Main Cluster Out"=w317:T5)  [unwired: 9 in]
                n139 = Bundle By Name(cluster=w317, "White Balance"=w313) -> (w314:T5)
              }
              event "VideoMode": Value Change {
                w318 = u16 20 items=["160x120 MJPG 30.00fps", "160x120 YUY2 30.00fps", "176x144 MJPG 30.00fps", "176x144 YUY2 30.00fps", "320x240 MJPG 30.00fps", "320x240 YUY2 30.00fps", "352x288 MJPG 30.00fps", "352x288 YUY2 30.00fps", "416x240 MJPG 30.00fps", "424x240 YUY2 30.00fps", "640x360 MJPG 30.00fps", "640x360 YUY2 30.00fps", "640x480 MJPG 30.00fps", "640x480 YUY2 30.00fps", "800x448 MJPG 30.00fps", "800x448 YUY2 20.00fps", "800x600 MJPG 30.00fps", "800x600 YUY2 15.00fps", "960x544 MJPG 30.00fps", "960x544 YUY2 15.00fps", "1280x720 MJPG 30.00fps", "1280x720 YUY2 10.00fps", "1280x800 YUY2 10.00fps"] ("VideoMode")
                w322 = T6 [enum."End Session", enum."Open Camera", enum."Get Values", enum."Setup Camera", enum."Start Session", enum."Get Values"] items=["Message Dispatcher", "INI", "End Session", "Camera Process Settings", "Camera Open Default", "Camera Save Default", "Get Values", "Get VideoMode", "Open Camera", "Open Settings", "Save Settings", "Set Value", "Set VideoMode", "Set WB", "Setup Camera", "Start Session", "Exit"] ("Main Queue")
                n140 = event-data() -> ("NewVal"=w320:u16)  [unwired: 1 in]
                n141 = Variant To Data(type=w318, Variant=w320) -> (data=w319:u16)  [unwired: 1 in, 1 out]
                n142 = Bundle By Name(cluster=w325, "VideoMode"=w319) -> (w324:T5)
                n143 = call "Main Add to Queue.vi"("Main Queue"=w322, "Main Cluster In"=w324) -> ("Main Cluster Out"=w323:T5)  [unwired: 9 in]
              }
            }
          }
          frame "INI" {
            # "We set up all of the values to the default value. You can change these values based on the cameras that you are using as well as different envionemntal conditions that my exist in your location."
            n144 = Unbundle By Name(w327) -> ("Open And Save Controls"=w326:refnum<vi>[])
            n145 = for {
              tunnel: w326 -> [w332] mode=indexing
              tunnel: [w331] -> w329 mode=indexing
              n146 = property class="Num"(reference=w332) -> ("Label.Text"=w331:string)  [unwired: 1 in, 2 out]
            }
            n147 = Bundle By Name(cluster=w327, "Attr String"=w329) -> (w328:T5)
          }
          frame "End Session" {
            # "This state will end the camera session"
            n148 = Unbundle By Name(w339) -> ("Camera Session"=w338:T8, "error"=w334:errorcluster)
            n149 = call <vilib>:"IMAQdx Close Camera.vi"("error in"=w334, "Session In"=w338) -> ("error out"=w333:errorcluster)  [unwired: 9 in]
            n150 = call <vilib>:"Clear Errors.vi"("error in (no error)"=w333) -> ("error out"=w335:errorcluster)  [unwired: 5 in, 1 out]
            n151 = Bundle By Name(cluster=w339, "error"=w335) -> (w336:T5)
          }
          frame "Camera Open Default" {
            # "This code opens a setup file that is used to save user preferences."
            n152 = Unbundle By Name(w347) -> ("Main Open and Save Ctrls Ref"=w340:refnum<vi>[], "Open And Save Controls"=w345:refnum<vi>[], "Camera"=w341:T8, "Default path"=w346:path)
            n153 = call "Attached Camera Info AE.vi"("InterfaceName"=w341) -> ("Serial Number"=w342:string)  [unwired: 10 in]
            n154 = call <vilib>:"Open Config Data.vi"("configuration file path"=w346) -> ("refnum"=w350:T11)  [unwired: 8 in, 2 out]
            n155 = for {
              tunnel: w350 -> [w367]
              tunnel: w342 -> [w353]
              tunnel: w345 -> [w366] mode=indexing
              tunnel: [w363] -> w348
              tunnel: [w361] -> w349
              tunnel: w340 -> [w359] mode=indexing
              n156 = property class="Num"(reference=w366) -> (reference out=w365:refnum<vi>, error out=w358:errorcluster, "Label.Text"=w357:string, "Value"=w360:variant)  [unwired: 1 in]
              n157 = Variant To Flattened String(Variant=w360) -> (data string=w354:string, 1:w356:i16[])
              n158 = call-poly <vilib>:"Read Key.vi"("section"=w353, "default value"=w354, "key"=w357, "refnum"=w367) -> ("error out"=w362:errorcluster, "value"=w352:string, "found?"=w355:bool, "refnum out"=w364:T11)  [unwired: 4 in]
              n159 = case shown="True" w355 {
                tunnel: w352 -> [_ w381]
                tunnel: w365 -> [_ w386]
                tunnel: w358 -> [_ w385]
                tunnel: w364 -> [w379 w384]
                tunnel: w353 -> [w378 _]
                tunnel: w357 -> [w377 _]
                tunnel: [w376 w384] -> w363
                tunnel: w362 -> [w375 w383]
                tunnel: [w374 w383] -> w361
                tunnel: w354 -> [w373 _]
                tunnel: w356 -> [_ w382]
                frame False {
                  n160 = call-poly <vilib>:"Write Key.vi"("section"=w378, "error in (no error)"=w375, "value"=w373, "key"=w377, "refnum"=w379) -> ("error out"=w374:errorcluster, "refnum out"=w376:T11)  [unwired: 4 in, 1 out]
                }
                frame True {
                  n161 = Flattened String To Variant(6:w381, 7:w382) -> (3:w380:variant)  [unwired: 1 in, 1 out]
                  n162 = property class="Num"(reference=w386, error in=w385, "Value"=w380) -> ()  [unwired: 2 out]
                }
              }
              n163 = case shown="True" w355 {
                tunnel: w352 -> [_ w369]
                tunnel: w359 -> [_ w372]
                tunnel: w358 -> [_ w371]
                tunnel: w356 -> [_ w370]
                frame False {
                }
                frame True {
                  n164 = Flattened String To Variant(6:w369, 7:w370) -> (3:w368:variant)  [unwired: 1 in, 1 out]
                  n165 = property class="Num"(reference=w372, error in=w371, "Value"=w368) -> ()  [unwired: 2 out]
                }
              }
            }
            n166 = call <vilib>:"Close Config Data.vi"("error in (no error)"=w349, "refnum"=w348) -> ()  [unwired: 8 in, 2 out]
            n167 = call "Stall Data Flow.vim"("value in"=w347, "milliseconds to wait"=u32 100) -> ("value out"=w344:T5)  [unwired: 1 out]
          }
          frame "Camera Process Settings" {
            w387 = T6 [enum."Set WB", enum."Set Value"] items=["Message Dispatcher", "INI", "End Session", "Camera Process Settings", "Camera Open Default", "Camera Save Default", "Get Values", "Get VideoMode", "Open Camera", "Open Settings", "Save Settings", "Set Value", "Set VideoMode", "Set WB", "Setup Camera", "Start Session", "Exit"] ("Main Queue")
            # "This event finds the cameras that I am looking for and get the alias name for the camera. You can do this any way you want to. This is an easy system that is bult into LabVIEW.  I look for the camera name I am looking for and send the alias on so the camera session can be set up."
            n168 = Bundle By Name(cluster=w390, "error"=errorcluster {"status"=FALSE, "code"=0, "source"=""}, "Main Queue"=w387) -> (w388:T5)
          }
          frame "Camera Save Default" {
            # "We save the camera setting that are important to a file so we can recall them later. The save function can be called anywhere this system is being used within the vision computer using the event fire. This can be found in frame zero of this code in the diable diagram."
            n169 = Unbundle By Name(w395) -> ("Camera"=w392:T8, "Default path"=w394:path, "Open And Save Controls"=w393:refnum<vi>[])
            n170 = call <vilib>:"Open Config Data.vi"("configuration file path"=w394) -> ("error out"=w396:errorcluster, "refnum"=w399:T11)  [unwired: 8 in, 1 out]
            n171 = for {
              tunnel: w393 -> [w408] mode=indexing
              tunnel: w399 -> [w410]
              tunnel: w392 -> [w409]
              tunnel: [w405] -> w398
              tunnel: [w403] -> w397
              tunnel: w396 -> [w402]
              n172 = property class="Num"(reference=w408, error in=w402) -> (error out=w404:errorcluster, "Label.Text"=w407:string, "Value"=w406:variant)  [unwired: 1 out]
              n173 = Variant To Flattened String(Variant=w406) -> (data string=w401:string)  [unwired: 1 out]
              n174 = call-poly <vilib>:"Write Key.vi"("section"=w409, "error in (no error)"=w404, "value"=w401, "key"=w407, "refnum"=w410) -> ("error out"=w403:errorcluster, "refnum out"=w405:T11)  [unwired: 4 in, 1 out]
            }
            n175 = call <vilib>:"Close Config Data.vi"("error in (no error)"=w397, "refnum"=w398) -> ()  [unwired: 8 in, 2 out]
          }
          frame "Get Values" {
            # "This step gets all the current setting in the camera if an INI file does not exist."
            n176 = Unbundle By Name(w417) -> ("Open And Save Controls"=w415:refnum<vi>[], "Camera Session"=w414:T8, "Attr String"=w418:string[], "error"=w421:errorcluster, "Main Open and Save Ctrls Ref"=w412:refnum<vi>[])
            n177 = for {
              N: 8 -> [_]
              tunnel: w418 -> [w436] mode=indexing
              shift-right: [w431] -> w420
              shift-left: w421 -> [w437]
              shift-right: [w435] -> w419
              shift-left: w414 -> [w438]
              tunnel: w415 -> [w433] mode=indexing
              tunnel: [w425] -> w413 mode=indexing
              tunnel: w412 -> [w427] mode=indexing
              n178 = call "CameraGetScaledAttrSharpness.vi"("error in (no error)"=w437, "Attr String"=w436, "IMAQdx Session"=w438) -> ("error out"=w434:errorcluster, "Scaled"=w425:dbl, "IMAQdx Session out"=w435:T8, "Max"=w424:dbl, "MinDBL"=w423:dbl)  [unwired: 3 in, 1 out]
              n179 = call <vilib>:"Clear Errors.vi"("error in (no error)"=w434) -> ("error out"=w432:errorcluster)  [unwired: 5 in, 1 out]
              n180 = Not A Number/Path/Refnum?(number/path/refnum=w425) -> (NaN/Path/Refnum?=w428:bool)
              n181 = Select(t=T10."Disabled and Grayed Out" ("Disabled"), s=w428, f=T10."Enabled" ("Disabled")) -> (s? t:f=w426:T10)
              n182 = property class="Num"(reference=w433, error in=w432, "Value"=w425, "DisabledEnum"=w426, "Maximum"=w424, "Minimum"=w423) -> (error out=w431:errorcluster)  [unwired: 1 out]
              n183 = property class="Num"(reference=w427, "Value"=w425, "DisabledEnum"=w426, "Maximum"=w424, "Minimum"=w423) -> ()  [unwired: 1 in, 2 out]
            }
            n184 = Bundle By Name(cluster=w417, "Values"=w413, "Camera Session"=w419, "error"=w420) -> (w416:T5)
          }
          frame "Get VideoMode" {
            # "This frame sets the frame rate and picture size for the different camera models."
            n185 = Unbundle By Name(w465) -> ("Camera Session"=w467:T8, "error"=w466:errorcluster, "Main Timeout ref"=w442:refnum<vi>)
            n186 = call "CameraSetModeAttr.vi"("error in"=w466, "Attr String"="VideoMode", "IMAQdx Session In"=w467) -> ("error out"=w459:errorcluster, "IMAQdx Session out"=w462:T8)  [unwired: 7 in]
            n187 = property class="IMAQdx"(reference=w462, error in=w459) -> (reference out=w461:T8, error out=w460:errorcluster, "VideoMode"=w440:u32)
            n188 = property on="VideoMode" class="Ring (strict)"() -> ("Strings []"=w458:string[])  [unwired: 2 in, 2 out]
            n189 = local write "VideoMode"(w440) -> ()
            n190 = call <vilib>:"Clear Errors.vi"("error in (no error)"=w460) -> ("error out"=w451:errorcluster)  [unwired: 5 in, 1 out]
            n191 = Index Array(array=w458, index=w440) -> (element=w457:string)
            n192 = Bundle By Name(cluster=w465, "Camera Session"=w461, "error"=w451) -> (w464:T5)
            n193 = control-ref of="VideoMode"() -> (w441:refnum<vi>)
            n194 = xnode "Match Regular Expression"("input string"=w457, "regular expression"="\\d++(\\.\\d{2})") -> ("whole match"=w455:string)  [unwired: 4 in, 4 out]
            n195 = property class="Ring (strict)"(reference=w441, "Value"=w440) -> ()  [unwired: 1 in, 2 out]
            n196 = Fract/Exp String To Number(string=w455, default (0 dbl)=u32 0 ("default (0 DBL)")) -> (number=w448:u32)  [unwired: 2 in, 1 out]
            n197 = Equal To 0?(x=w448) -> (x = 0?=w449:bool)
            n198 = Select(t=u32 10, s=w449, f=w448) -> (s? t:f=w445:u32)
            n199 = Reciprocal(x=w445) -> (1/x=w454:dbl)
            n200 = Multiply(x=w454, y=u32 1000) -> (x*y=w453:dbl)
            n201 = To Unsigned Long Integer(number=w453) -> (unsigned 32bit integer=w446:u32)
            n202 = Decrement(x=w446) -> (x-1=w443:u32)
            n203 = Subtract(x=w443, y=u32 2) -> (x-y=w439:u32)
            n204 = property class="DigNum (strict)"(reference=w442, "Value"=w439) -> ()  [unwired: 1 in, 2 out]
            n205 = local write "Timeout"(w439) -> ()
          }
          frame "Open Camera" {
            n206 = Unbundle By Name(w591) -> ("Camera"=w588:T8)
            n207 = call <vilib>:"IMAQdx Open Camera.vi"("error in"=errorcluster {"status"=FALSE, "code"=0, "source"=""}, "Session In"=w588) -> ("error out"=w587:errorcluster, "Session Out"=w592:T8)  [unwired: 8 in]
            n208 = Bundle By Name(cluster=w591, "Camera Session"=w592, "error"=w587) -> (w590:T5)
            n209 = call <vilib>:"IMAQdx Enumerate Video Modes.vi"("Session In"=w592) -> ("error out"=w593:errorcluster, "Video Modes"=w594:T12)  [unwired: 7 in, 2 out]
            n210 = call <vilib>:"Clear Errors.vi"("error in (no error)"=w593) -> ()  [unwired: 5 in, 2 out]
            n211 = for {
              tunnel: w594 -> [w598] mode=indexing
              tunnel: [w597] -> w586 mode=indexing
              n212 = Unbundle By Name(w598) -> ("Video Mode Name"=w597:string)
            }
            n213 = property on="VideoMode" class="Ring (strict)"("Strings []"=w586) -> ()  [unwired: 2 in, 2 out]
            n214 = call "Event Generate Event.vi"("Camera Name"=w585, "Video Modes"=w586, "Event Type"=Event_Setup_Types."Update Video Mode") -> ()  [unwired: 9 in]
          }
          frame "Open Settings" {
            # "This code opens a setup file that is used to save user preferences."
            n215 = Unbundle By Name(w610) -> ("Main Open and Save Ctrls Ref"=w601:refnum<vi>[], "Open And Save Controls"=w608:refnum<vi>[], "Camera"=w607:T8, "INI path"=w609:path)
            n216 = call <vilib>:"Open Config Data.vi"("configuration file path"=w609) -> ("refnum"=w613:T11)  [unwired: 8 in, 2 out]
            n217 = for {
              tunnel: w613 -> [w632]
              tunnel: w607 -> [w628]
              tunnel: w608 -> [w631] mode=indexing
              tunnel: [w627] -> w611
              tunnel: [w625] -> w612
              tunnel: [w619] -> _ mode=indexing
              tunnel: [w622] -> w605 mode=indexing
              tunnel: [w621] -> w602 mode=indexing
              tunnel: w601 -> [w620] mode=indexing
              n218 = property class="Num"(reference=w631) -> (reference out=w630:refnum<vi>, error out=w616:errorcluster, "Label.Text"=w621:string, "Value"=w624:variant)  [unwired: 1 in]
              n219 = Variant To Flattened String(Variant=w624) -> (data string=w623:string, 1:w617:i16[])
              n220 = call-poly <vilib>:"Read Key.vi"("section"=w628, "default value"=w623, "key"=w621, "refnum"=w632) -> ("error out"=w626:errorcluster, "value"=w618:string, "found?"=w619:bool, "refnum out"=w629:T11)  [unwired: 4 in]
              n221 = case shown="True" w619 {
                tunnel: w618 -> [_ w649]
                tunnel: w630 -> [_ w654]
                tunnel: w616 -> [_ w653]
                tunnel: w629 -> [w647 w652]
                tunnel: w628 -> [w646 _]
                tunnel: w621 -> [w645 _]
                tunnel: [w644 w652] -> w627
                tunnel: w626 -> [w643 w651]
                tunnel: [w642 w651] -> w625
                tunnel: w623 -> [w641 _]
                tunnel: w617 -> [_ w650]
                tunnel: [variant ("Variant") w648] -> w622
                frame False {
                  n222 = call-poly <vilib>:"Write Key.vi"("section"=w646, "error in (no error)"=w643, "value"=w641, "key"=w645, "refnum"=w647) -> ("error out"=w642:errorcluster, "refnum out"=w644:T11)  [unwired: 4 in, 1 out]
                }
                frame True {
                  n223 = Flattened String To Variant(6:w649, 7:w650) -> (3:w648:variant)  [unwired: 1 in, 1 out]
                  n224 = property class="Num"(reference=w654, error in=w653, "Value"=w648) -> ()  [unwired: 2 out]
                }
              }
              n225 = case shown="True" w619 {
                tunnel: w620 -> [w633 w639]
                tunnel: w616 -> [_ w638]
                tunnel: w617 -> [_ w637]
                tunnel: [w633 w635] -> _
                tunnel: w618 -> [_ w634]
                frame False {
                }
                frame True {
                  n226 = Flattened String To Variant(6:w634, 7:w637) -> (3:w636:variant)  [unwired: 1 in, 1 out]
                  n227 = property class="Num"(reference=w639, error in=w638, "Value"=w636) -> (reference out=w635:refnum<vi>)  [unwired: 1 out]
                }
              }
            }
            n228 = call <vilib>:"Close Config Data.vi"("error in (no error)"=w612, "refnum"=w611) -> ()  [unwired: 8 in, 2 out]
            n229 = Variant To Data(type=dbl[] [], Variant=w605) -> (data=w604:dbl[], error out=w599:errorcluster)  [unwired: 1 in]
            n230 = flat-sequence {
              tunnel: [w615] -> w600
              tunnel: w599 -> [_]
              frame #0 {
                n231 = local read "VideoMode"() -> (w615:u16)
              }
            }
            n232 = Bundle By Name(cluster=w610, "Attr String"=w602, "Values"=w604, "VideoMode"=w600) -> (w606:T5)
          }
          frame "Save Settings" {
            # "We save the camera setting that are important to a file so we can recall them later. The save function can be called anywhere this system is being used within the vision computer using the event fire. This can be found in frame zero of this code in the diable diagram."
            n233 = Unbundle By Name(w658) -> ("Camera"=w655:T8, "INI path"=w657:path, "Open And Save Controls"=w656:refnum<vi>[])
            n234 = call <vilib>:"Open Config Data.vi"("configuration file path"=w657) -> ("error out"=w659:errorcluster, "refnum"=w662:T11)  [unwired: 8 in, 1 out]
            n235 = for {
              tunnel: w656 -> [w671] mode=indexing
              tunnel: w662 -> [w673]
              tunnel: w655 -> [w672]
              tunnel: [w668] -> w661
              tunnel: [w666] -> w660
              tunnel: w659 -> [w665]
              n236 = property class="Num"(reference=w671, error in=w665) -> (error out=w667:errorcluster, "Label.Text"=w670:string, "Value"=w669:variant)  [unwired: 1 out]
              n237 = Variant To Flattened String(Variant=w669) -> (data string=w664:string)  [unwired: 1 out]
              n238 = call-poly <vilib>:"Write Key.vi"("section"=w672, "error in (no error)"=w667, "value"=w664, "key"=w670, "refnum"=w673) -> ("error out"=w666:errorcluster, "refnum out"=w668:T11)  [unwired: 4 in, 1 out]
            }
            n239 = call <vilib>:"Close Config Data.vi"("error in (no error)"=w660, "refnum"=w661) -> ()  [unwired: 8 in, 2 out]
          }
          frame "Set Value" {
            # "This frame sets the frame rate and picture size for the different camera models."
            n240 = Unbundle By Name(w677) -> ("Camera Session"=w682:T8, "Attr String"=w675:string[], "error"=w681:errorcluster, "Values"=w678:dbl[])
            n241 = for {
              N: 8 -> [_]
              tunnel: w678 -> [w684] mode=indexing
              tunnel: w675 -> [w686] mode=indexing
              shift-right: [w687] -> w680
              shift-left: w681 -> [w690]
              shift-right: [w688] -> w679
              shift-left: w682 -> [w692]
              n242 = call "CameraSetModeAttr.vi"("error in"=w690, "Attr String"=w686, "IMAQdx Session In"=w692) -> ("error out"=w689:errorcluster, "IMAQdx Session out"=w691:T8)  [unwired: 7 in]
              n243 = call "CameraSetScaledAttr.vi"("error in"=w689, "Scaled"=w684, "Attr String"=w686, "IMAQdx Session in"=w691) -> ("error out"=w685:errorcluster, "IMAQdx Session"=w688:T8)  [unwired: 6 in]
              n244 = call <vilib>:"Clear Errors.vi"("error in (no error)"=w685) -> ("error out"=w687:errorcluster)  [unwired: 5 in, 1 out]
            }
            n245 = Bundle By Name(cluster=w677, "Camera Session"=w679, "error"=w680) -> (w676:T5)
          }
          frame "Set WB" {
            w703 = 0.0 ("Color Temp (K)")
            # "Here is where you set the White Balance for the camera. We also notify the NT table so the control on the processing software and dashboard can be updated if something is changed in this software. By sending this to the NT table we keep everything syncronized."
            n246 = Unbundle By Name(w695) -> ("Camera Session"=w699:T8, "error"=w696:errorcluster, "White Balance"=w693:T2)
            n247 = call "CameraWhiteBalanceConstants.vi"() -> ("Color Temps (K)"=w702:dbl[])  [unwired: 11 in]
            n248 = Build Array (concatenate)(w702, w703, w703) -> (w701:dbl[])
            n249 = case shown="Default" w693 {
              selector: w693 -> [w716 w725]
              tunnel: w701 -> [w717 _]
              tunnel: "CameraAttributes::WhiteBalance::Value" -> [w714 _]
              tunnel: [w712 w719] -> w697
              tunnel: w699 -> [w710 w723]
              tunnel: "WhiteBalance" -> [w709 w722]
              tunnel: [w708 w720] -> w698
              tunnel: w696 -> [w707 w718]
              frame Default {
                n250 = Decrement(x=w716) -> (x-1=w715:T2)
                n251 = call "CameraSetModeAttr.vi"("error in"=w707, "Attr String"=w709, "IMAQdx Session In"=w710) -> ("error out"=w706:errorcluster, "IMAQdx Session out"=w711:T8)  [unwired: 7 in]
                n252 = Index Array(array=w717, index=w715) -> (element=w713:dbl)
                n253 = property class="IMAQdx"(reference=w711, error in=w706, "ActiveAttribute"=w714, "ValueDBL"=w713) -> (reference out=w708:T8, error out=w712:errorcluster)
              }
              frame "Auto", "Hold current" {
                n254 = Equal To 0?(x=w725) -> (x = 0?=w724:bool)
                n255 = Select(t="Auto", s=w724, f="Manual") -> (s? t:f=w721:string)
                n256 = call "CameraSetModeAttr.vi"("error in"=w718, "Value"=w721, "Attr String"=w722, "IMAQdx Session In"=w723) -> ("error out"=w719:errorcluster, "IMAQdx Session out"=w720:T8)  [unwired: 6 in]
              }
            }
            n257 = Bundle By Name(cluster=w695, "Camera Session"=w698, "error"=w697) -> (w705:T5)
          }
          frame "Setup Camera" {
            # "Reg Ex to find the frame rate so we can adjust the loop speed."
            # "This state sets up the placeholder for the camera image."
            n258 = Unbundle By Name(w754) -> ("Camera Session"=w729:T8, "VideoMode"=w730:u16, "Main Timeout ref"=w732:refnum<vi>)
            n259 = property class="IMAQdx"(reference=w729, "VideoMode"=w730) -> (reference out=w736:T8, error out=w735:errorcluster)  [unwired: 1 in]
            n260 = call "IMAQ Create"("Border Size"=0, "Image Name"=w729) -> ("New Image"=w750:T1)  [unwired: 3 in, 1 out]
            n261 = control-ref of="VideoMode"() -> (w731:refnum<vi>)
            n262 = property class="Ring (strict)"(reference=w731, "Value"=w730) -> ()  [unwired: 1 in, 2 out]
            n263 = Bundle By Name(cluster=w754, "Camera Session"=w736, "error"=w735, "Image In"=w750) -> (w753:T5)
            n264 = property on="VideoMode" class="Ring (strict)"("Value"=w730) -> ("Strings []"=w733:string[])  [unwired: 2 in, 2 out]
            n265 = case shown="No Error" w735 {
              tunnel: w753 -> [w872 w875]
              tunnel: [w872 w874] -> w752
              frame No Error {
              }
              frame Error {
                w873 = T6 [] items=["Message Dispatcher", "INI", "End Session", "Camera Process Settings", "Camera Open Default", "Camera Save Default", "Get Values", "Get VideoMode", "Open Camera", "Open Settings", "Save Settings", "Set Value", "Set VideoMode", "Set WB", "Setup Camera", "Start Session", "Exit"] ("Main Queue")
                # "Clear the queue"
                n266 = Bundle By Name(cluster=w875, "Main Queue"=w873) -> (w874:T5)
              }
            }
            n267 = Index Array(array=w733, index=w730) -> (element=w749:string)
            n268 = xnode "Match Regular Expression"("input string"=w749, "regular expression"="\\d++(\\.\\d{2})") -> ("whole match"=w747:string)  [unwired: 4 in, 4 out]
            n269 = Fract/Exp String To Number(string=w747, default (0 dbl)=u32 0 ("default (0 DBL)")) -> (number=w741:u32)  [unwired: 2 in, 1 out]
            n270 = Equal To 0?(x=w741) -> (x = 0?=w742:bool)
            n271 = Select(t=u32 10, s=w742, f=w741) -> (s? t:f=w739:u32)
            n272 = Reciprocal(x=w739) -> (1/x=w746:dbl)
            n273 = Multiply(x=w746, y=u32 1000) -> (x*y=w745:dbl)
            n274 = To Unsigned Long Integer(number=w745) -> (unsigned 32bit integer=w738:u32)
            n275 = Decrement(x=w738) -> (x-1=w737:u32)
            n276 = Subtract(x=w737, y=u32 2) -> (x-y=w728:u32)
            "Timeout" <- w728
            n277 = property class="DigNum (strict)"(reference=w732, "Value"=w728) -> ()  [unwired: 1 in, 2 out]
          }
          frame "Start Session" {
            w879 = u32 3 items=["Get Oldest"=0, "Fail"=2, "Get Newest"=3] ("OverwriteMode")
            # "This state starts the camera session and passes it to the rest of the code so it can be used. We also get the picture size."
            n278 = Unbundle By Name(w890) -> ("Camera Session"=w876:T8, "error"=w881:errorcluster, "INI File Found"=w877:bool)
            n279 = property class="IMAQdx"(reference=w876, error in=w881, "OverwriteMode"=w879) -> (reference out=w882:T8, error out=w880:errorcluster)
            n280 = call <vilib>:"IMAQdx Configure Grab.vi"("error in"=w880, "Session In"=w882) -> ("error out"=w888:errorcluster, "Session Out"=w886:T8)  [unwired: 8 in]
            n281 = property class="IMAQdx"(reference=w886, error in=w888) -> (error out=w889:errorcluster, "Height"=→"Height 2":u32, "Width"=→"Width 2":u32)  [unwired: 1 out]
            n282 = Bundle By Name(cluster=w890, "Camera Session"=w886, "error"=w889) -> (w885:T5)
            n283 = First Call?() -> (First Call?: T/F=w883:bool)
            n284 = And(x=w883, y=w877) -> (x .and. y?=w878:bool)
            n285 = case shown="True" w878 {
              tunnel: w885 -> [w893 w896]
              tunnel: [w893 w895] -> w884
              frame False {
              }
              frame True {
                w894 = T6 [enum."Camera Process Settings"] items=["Message Dispatcher", "INI", "End Session", "Camera Process Settings", "Camera Open Default", "Camera Save Default", "Get Values", "Get VideoMode", "Open Camera", "Open Settings", "Save Settings", "Set Value", "Set VideoMode", "Set WB", "Setup Camera", "Start Session", "Exit"] ("Main Queue")
                n286 = call "Main Add to Queue.vi"("Main Queue"=w894, "Main Cluster In"=w896) -> ("Main Cluster Out"=w895:T5)  [unwired: 9 in]
              }
            }
          }
          frame "Exit" {
            # "The end frame is where we shut this software down when we want to exit the program."
          }
        }
      }
    }
  }
  "Title" <- "Camera"
